vi "CRC16-CCITT Check (SubVI).vi"(11 "Data In (u8)":u8[](array[numeric])) -> (3 "CRC Calc":u16)   [LabVIEW 2019]
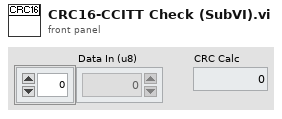
[diagram p1: front panel]
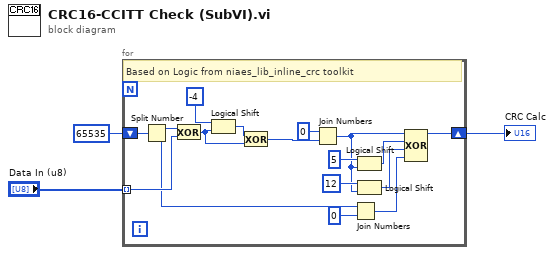
[diagram p0: block diagram]
diagram:
  n1 = for {
    shift-right: [w5] -> w1
    shift-left: u16 65535 ("Initial CRC") -> [w15]
    tunnel: "Data In (u8)" -> [w14] mode=indexing
    # "Based on Logic from niaes_lib_inline_crc toolkit"
    n2 = Split Number(x=w15) -> (hi(x)=w20:u8, lo(x)=w6:u8)
    n3 = Exclusive Or(1:w14, 2:w20) -> (0:w16:u8)
    n4 = Logical Shift(y=i8 -4, x=w16) -> (x << y=w4:u8)
    n5 = Exclusive Or(1:w16, 2:w4) -> (0:w18:u8)
    n6 = Join Numbers(hi=u8 0, lo=w18) -> ((hi.lo)=w7:u16)
    n7 = Join Numbers(hi=w6, lo=u8 0) -> ((hi.lo)=w8:u16)
    n8 = Logical Shift(y=i8 5, x=w7) -> (x << y=w12:u16)
    n9 = Logical Shift(y=i8 12, x=w7) -> (x << y=w10:u16)
    n10 = Compound Arithmetic op=XOR(w7, w12, w10, w8) -> (w5:u16)
  }
  "CRC Calc" <- w1
